vi "Try Match Response.vi"(8 "error in":errorcluster, 10 "ICAN CC Frame":refnum<class "ICAN CC Frame.lvclass">, 11 "Block Upload End Transfer in":refnum<class "Block Upload End Transfer.lvclass">) -> (0 "error out":errorcluster, 2 "Match":bool, 3 "SDO Transfer out":refnum<class "SDO Transfer.lvclass">)   [LabVIEW 2020, in "CANopen.lvlib" / "SDO Manager.lvlib" / "Block Upload End Transfer.lvclass"]
uses:
  Block Upload End Transfer.lvclass
  Block Upload End Transfer.lvclass/Block Upload End Transfer.ctl
  SDO Transfer/SDO Transfer.lvclass
  CANopen Message/CANopen Message.lvclass
  HAL/Source/Interfaces/ICAN CC Frame/ICAN CC Frame.lvclass
panel:
  out "number":u32
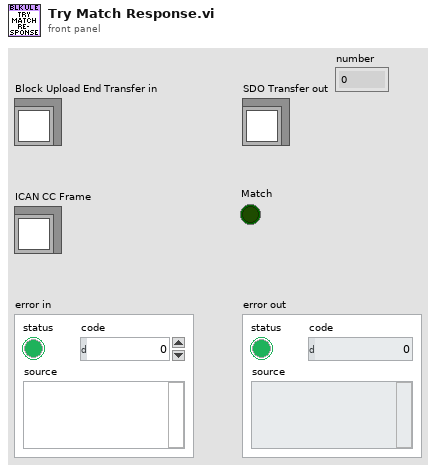
[diagram p1: front panel]
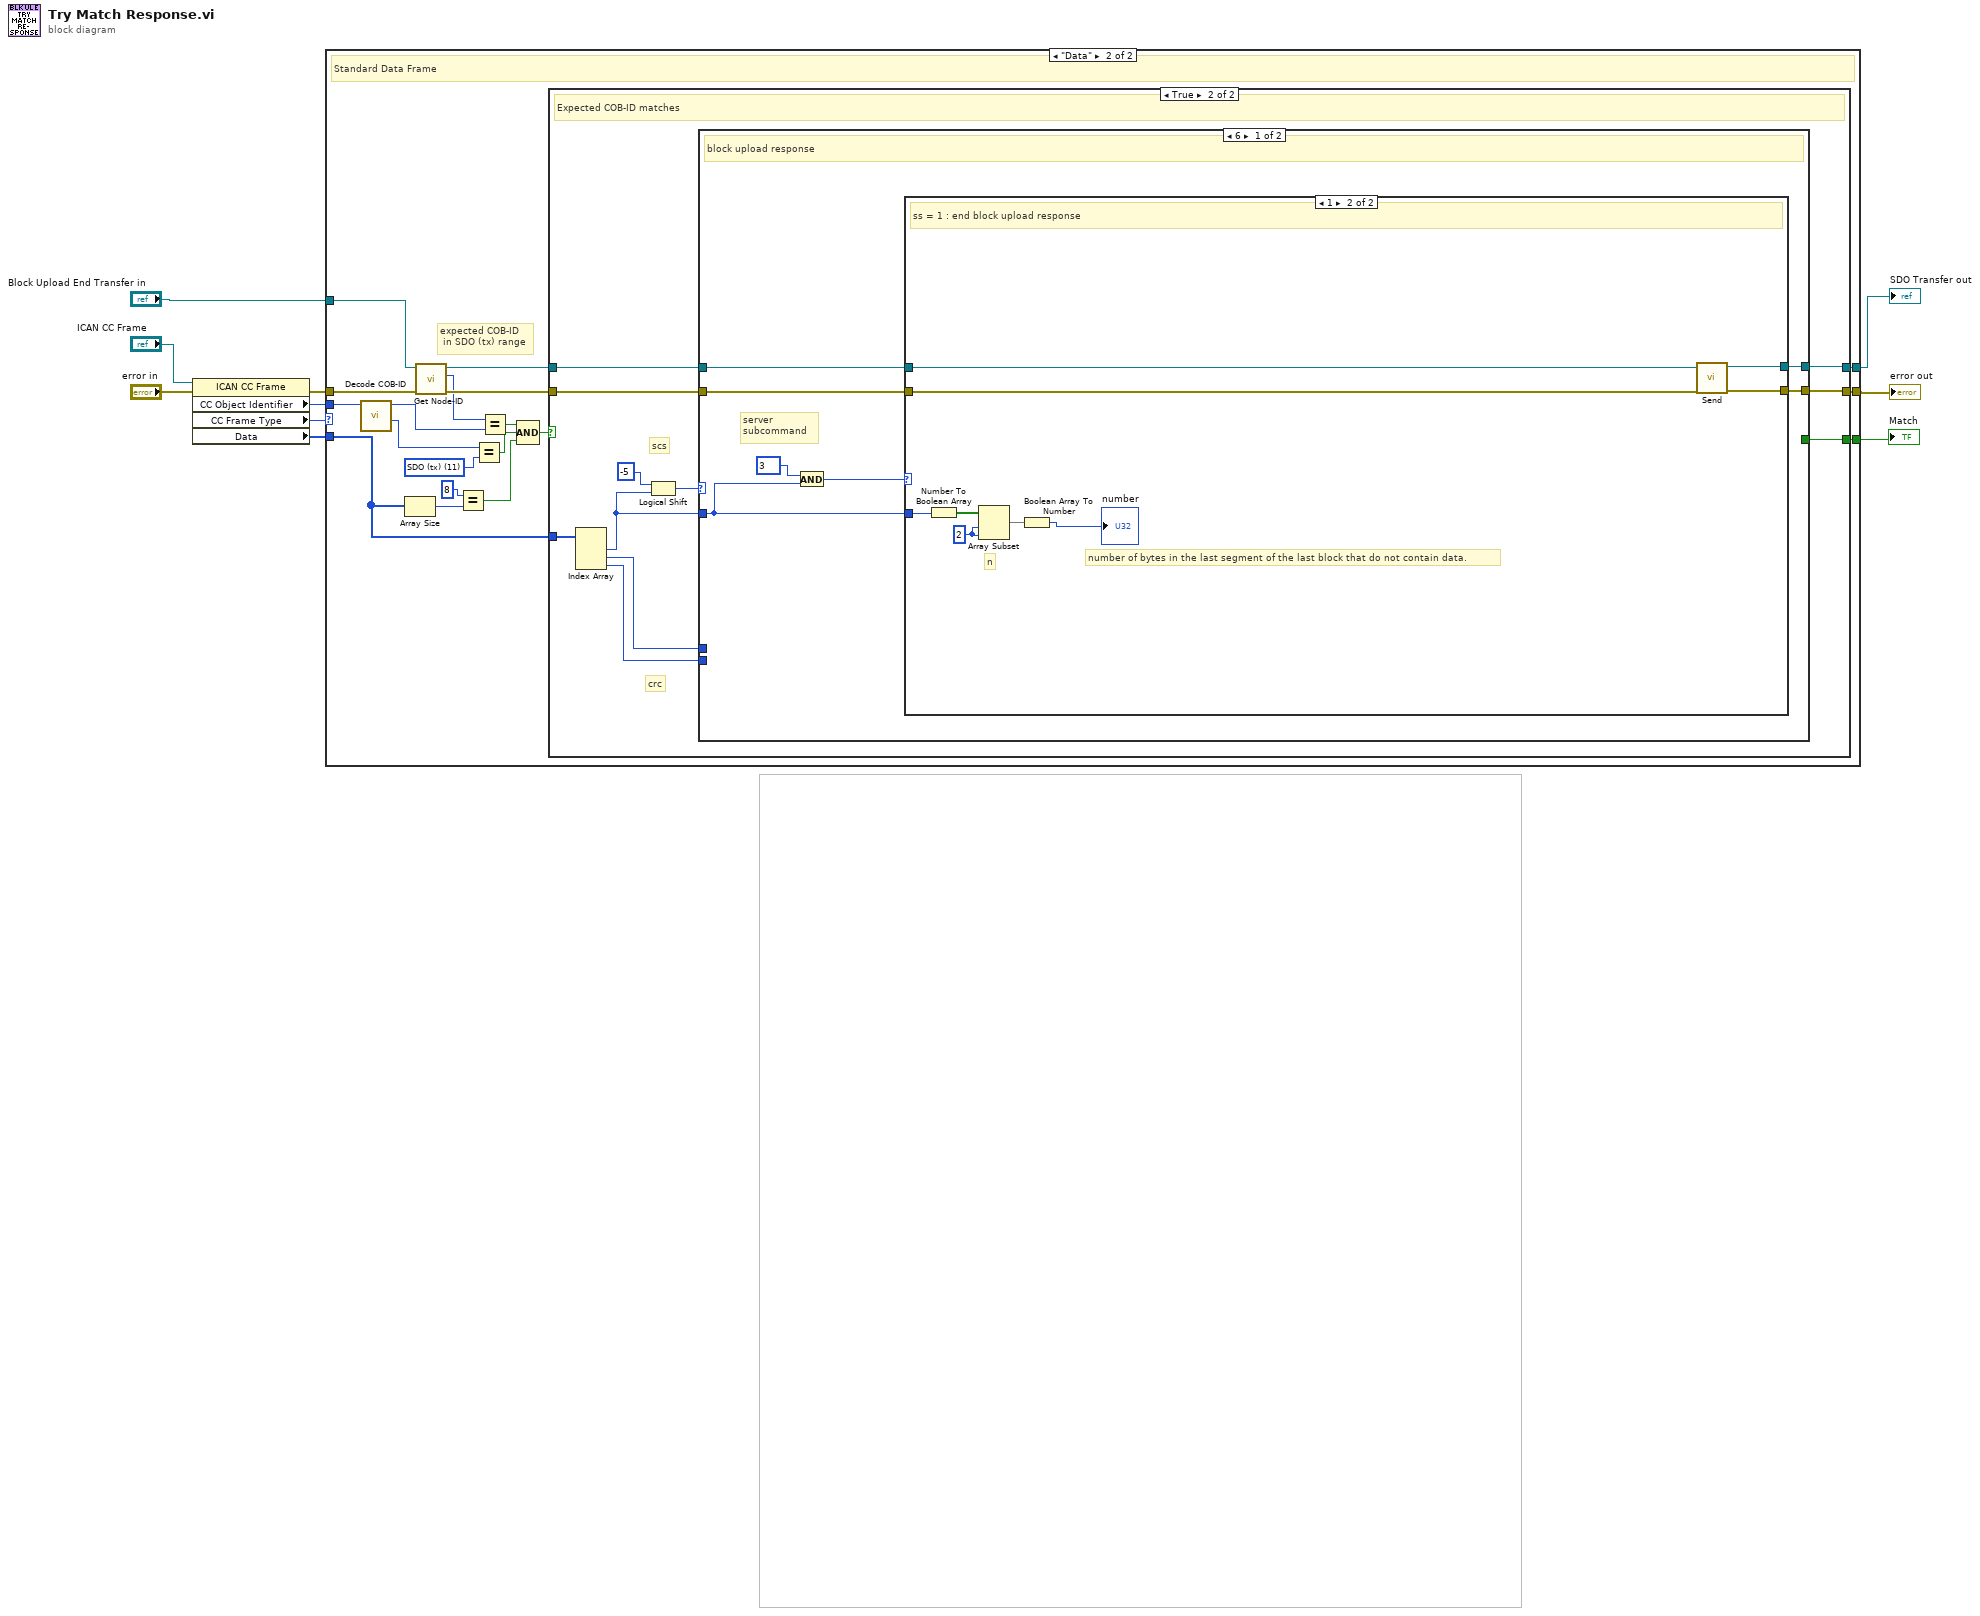
[diagram p0: block diagram]
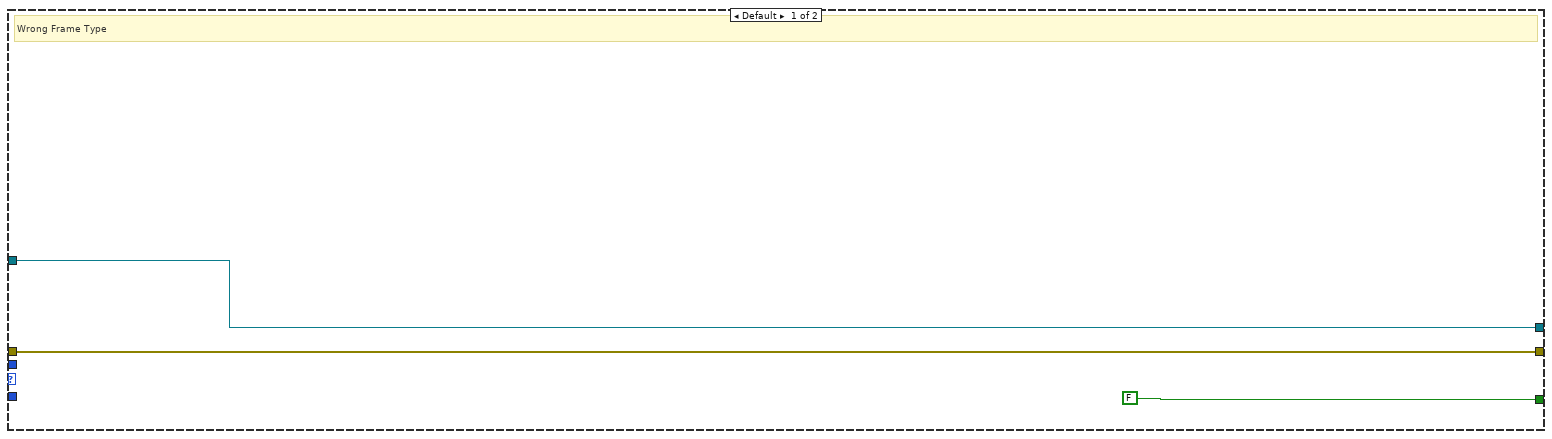
[diagram p2: hidden frame]
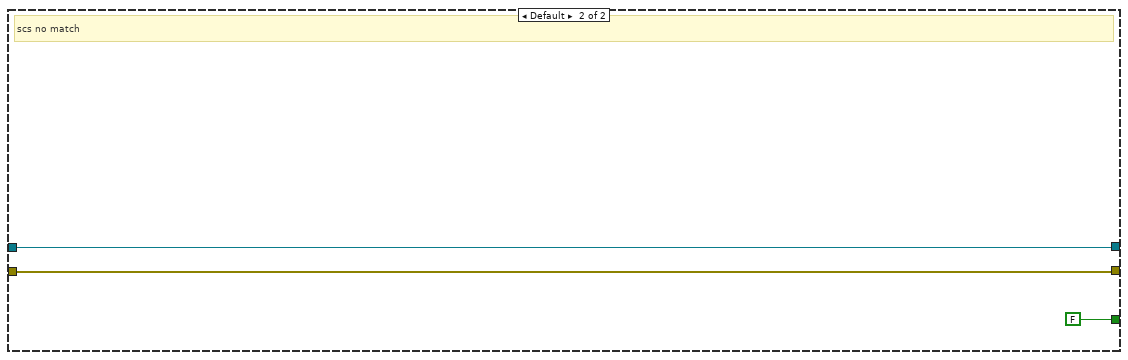
[diagram p5: hidden frame]
diagram:
  n1 = property class="ICAN CC Frame"(reference="ICAN CC Frame", error in="error in") -> (error out=w10:errorcluster, "CC Object Identifier"=w9:u32, "CC Frame Type"=w7:enum8{"Data", "Remote", "Error", "Overload"}, "Data"=w8:u8[])  [unwired: 1 out]
  n2 = case shown="\"Data\"" w7 {
    tunnel: w10 -> [w12 w32]
    tunnel: "Block Upload End Transfer in" -> [w11 w31]
    tunnel: [w11 w28] -> w4
    tunnel: [w12 w27] -> w6
    tunnel: [FALSE w26] -> w5
    tunnel: w9 -> [_ w25]
    tunnel: w8 -> [_ w14]
    frame Default {
      # "Wrong Frame Type"
    }
    frame "Data" {
      w22 = u8 11 items=["NMT"=0, "EMCY/SYNC"=1, "TIME"=2, "PDO1 (tx)"=3, "PDO1 (rx)"=4, "PDO2 (tx)"=5, "PDO2 (rx)"=6, "PDO3 (tx)"=7, "PDO3 (rx)"=8, "PDO4 (tx)"=9, "PDO4 (rx)"=10, "SDO (tx)"=11, "SDO (rx)"=12, "NMT error control"=14] ("Function Code")
      # "expected COB-ID\n in SDO (tx) range"
      # "Standard Data Frame"
      n3 = call "Decode COB-ID.vi"("COD-ID"=w25) -> ("Function Code"=w21:u8, "Node-ID"=w24:u8)  [unwired: 9 in]
      n4 = Array Size(array=w14) -> (size(s)=w20:i32)
      n5 = call "Get Node-ID.vi"("error in"=w32, "SDO Transfer in"=w31) -> ("error out"=w29:errorcluster, "Node-ID"=w23:u8, "SDO Transfer out"=w30:refnum<class "Block Upload End Transfer.lvclass">)  [unwired: 7 in]
      n6 = Equal?(x=8, y=w20) -> (x = y?=w15:bool)
      n7 = Equal?(x=w21, y=w22) -> (x = y?=w16:bool)
      n8 = Equal?(x=w23, y=w24) -> (x = y?=w17:bool)
      n9 = Compound Arithmetic op=AND(w17, w16, w15) -> (w18:bool)
      n10 = case shown="True" w18 {
        tunnel: w30 -> [w34 w44]
        tunnel: w29 -> [w33 w43]
        tunnel: [w34 w37] -> w28
        tunnel: [w33 w38] -> w27
        tunnel: w14 -> [_ w41]
        tunnel: [_ w36] -> w26
        frame False {
        }
        frame True {
          # "crc"
          # "scs"
          # "Expected COB-ID matches"
          n11 = Index Array(array=w41) -> (element #1=w35:u8, element #2=w40:u8, element #3=w39:u8)  [unwired: 3 in]
          n12 = Logical Shift(y=i16 -5, x=w35) -> (x << y=w42:u8)
          n13 = case shown="6" w42 {
            tunnel: w40 -> [_ _]
            tunnel: w39 -> [_ _]
            tunnel: w44 -> [w49 w65]
            tunnel: w43 -> [w48 w66]
            tunnel: [w46 w65] -> w37
            tunnel: [w47 w66] -> w38
            tunnel: [_ FALSE] -> w36
            tunnel: w35 -> [w50 _]
            frame 6 {
              # "server\nsubcommand"
              # "block upload response"
              n14 = And(x=u8 3, y=w50) -> (x .and. y?=w51:u8)
              n15 = case shown="1" w51 {
                tunnel: w50 -> [_ w63]
                tunnel: w49 -> [w53 w56]
                tunnel: w48 -> [w54 w57]
                tunnel: [w54 w59] -> w47
                tunnel: [w53 w58] -> w46
                frame 0, Default {
                  # "invalid server subcommand?"
                }
                frame 1 {
                  w61 = 2 ("index")
                  # "number of bytes in the last segment of the last block that do not contain data."
                  # "n"
                  # "ss = 1 : end block upload response"
                  n16 = Number To Boolean Array(number=w63) -> (Boolean array=w62:bool[])
                  n17 = Array Subset(array=w62, index=w61, length=w61) -> (w60:bool[])
                  n18 = Boolean Array To Number(Boolean array=w60) -> (number=→"number":u32)
                  n19 = call-dynamic "Send.vi"("error in"=w57, "Block Upload End Transfer in"=w56) -> ("error out"=w59:errorcluster, "Block Upload End Transfer out"=w58:refnum<class "Block Upload End Transfer.lvclass">)  [unwired: 8 in]
                }
              }
            }
            frame Default {
              # "scs no match"
            }
          }
        }
      }
    }
  }
  "SDO Transfer out" <- w4
  "error out" <- w6
  "Match" <- w5
